vi "Meu_IP_Address.vi"() -> (0 "Meu IP":string, 2 "Nome computador":string)   [LabVIEW 2019]
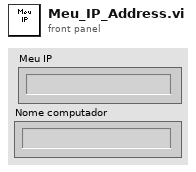
[diagram p1: front panel]
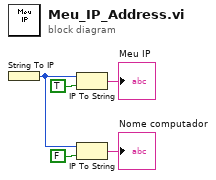
[diagram p0: block diagram]
diagram:
  n1 = String To IP() -> (0:w3:u32)  [unwired: 1 in]
  n2 = IP To String(1:TRUE ("dot notation? (F)"), 2:w3) -> (0:→"Meu IP":string)
  n3 = IP To String(1:FALSE ("dot notation? (F)"), 2:w3) -> (0:→"Nome computador":string)
